vi "Find SGP and PTP.vi"(8 "Error In":errorcluster, 9 "File Path":path, 10 "Pressure, Audio, EGG":dynamicdata(graph)) -> (0 "Error Out":errorcluster, 1 "File Path Indicator":path, 2 "PTP Array":dbl[](array[numeric]), 3 "SGP Array":dbl[](array[numeric]))   [LabVIEW 2018, in "AnalysisSupport.lvlib"]
uses:
  AnalysisSupport.lvlib
  Controls/Intervals.ctl
  <vilib>/Utility/miscctls.llb/LVCursorListTypeDef.ctl
  <vilib>/Waveform/WDTOps.llb/WDT Get XY Value DBL.vi
panel:
  out "PTP":dbl format="%#.3g"
  out "75ms Array":dbl[](array[numeric])
  out "150ms Array":dbl[](array[numeric])
  out "Cutoff (s)":dbl format="%#.3g"
  in  "Show EGG":bool
  in  "Show Audio":bool
  out "File Name":string
  out "End (s)":dbl format="%#.3g"
  out "+75ms":dbl format="%#.3g"
  out "Start (s)":dbl format="%#.3g"
  in  "Undo Button":bool
  in  "Interval (ms)":T1 items=["1000", "500", "330", "250", "150", "50"]
  out "Subset":dynamicdata(graph)
  out "Full Plot":dynamicdata(graph)
  out "Interruptions":i32
  out "SGP":dbl format="%#.3g"
  in  "Okay":bool
  in  "Mark Pressure":bool
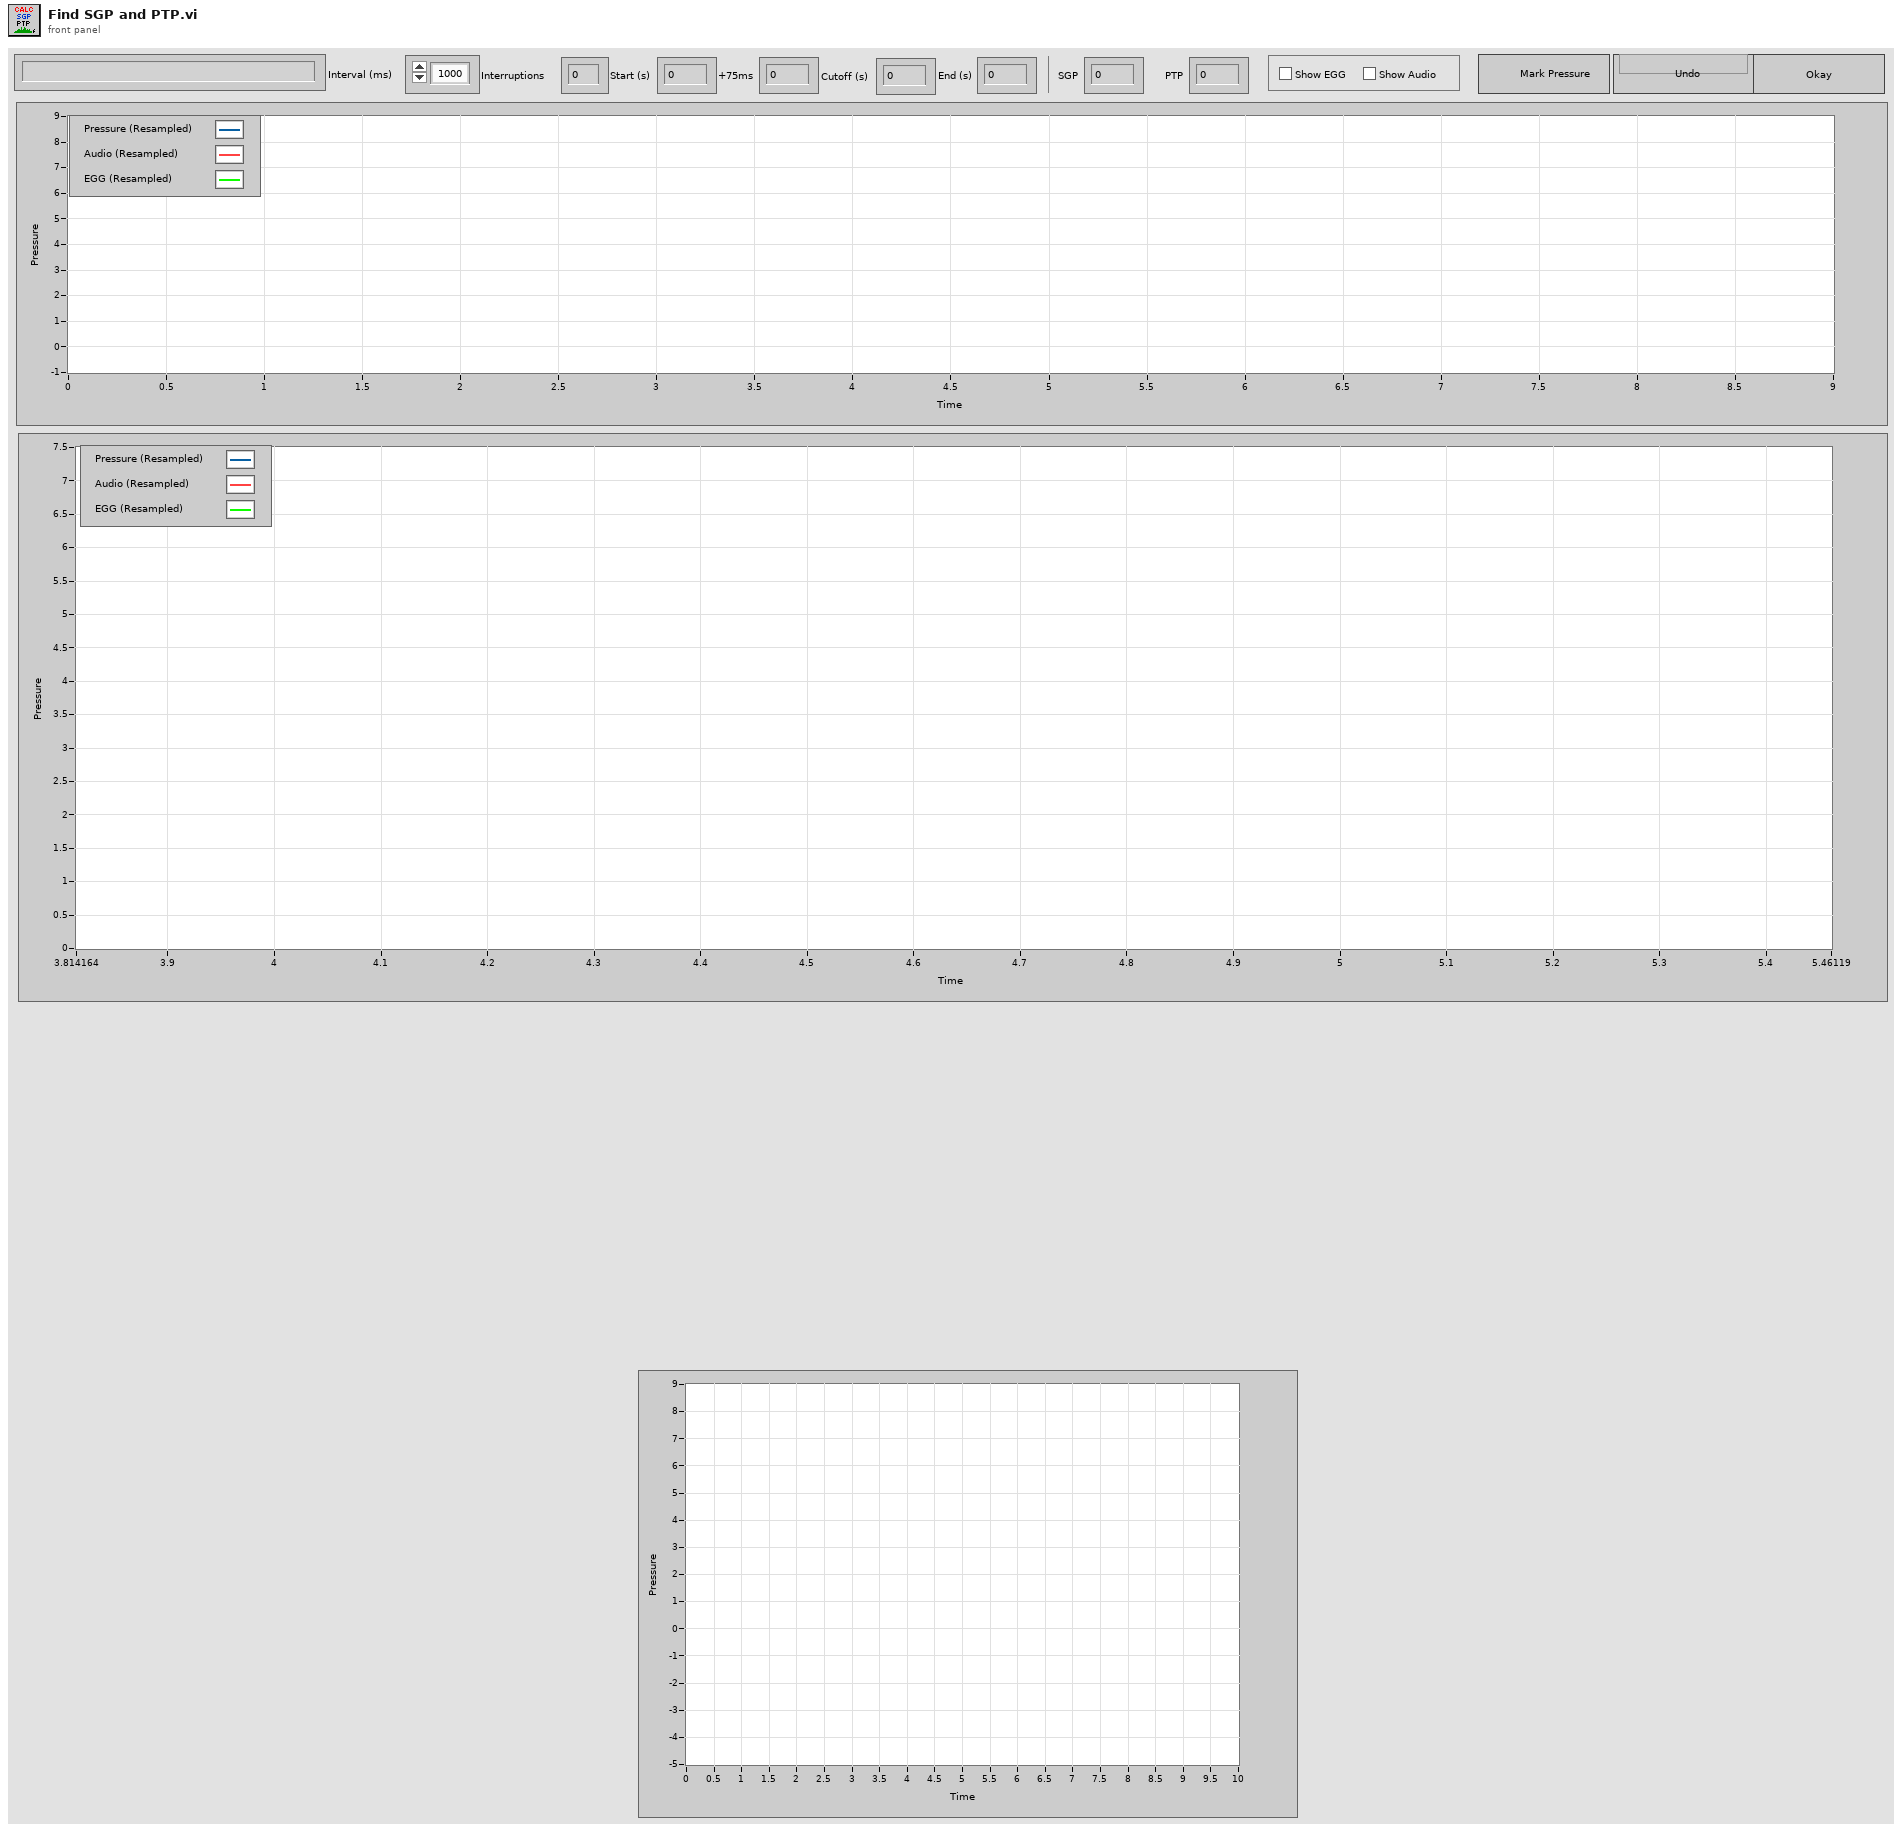
[diagram p1: front panel]
types:
  T1 = typedef "AnalysisSupport.lvlib/Intervals.ctl" = u16
  T2 = typedef "LVCursorListTypeDef.ctl" = cluster{"Name":string, "Color":u32, "Style":u8, "Point Style":u8, "Name Visible":bool, "Allow Drag":bool, "Cursor Mode":u32, "Plot":i32, "Index":i32, "Position":cluster{"X":dbl, "Y":dbl}, "X Scale":u32, "Y Scale":u32, "Watch Plots":i32[], "Watch All Plots":bool, "Plot Area":i32, "Label Offset":cluster{"X":dbl, "Y":dbl}}[]
  T3 = cluster{"Cursor List[0]":cluster{"Name":string, "Color":u32, "Style":u8, "Point Style":u8, "Name Visible":bool, "Allow Drag":bool, "Cursor Mode":u32, "Plot":i32, "Index":i32, "Position":cluster{"X":dbl, "Y":dbl}, "X Scale":u32, "Y Scale":u32, "Watch Plots":i32[], "Watch All Plots":bool, "Plot Area":i32, "Label Offset":cluster{"X":dbl, "Y":dbl}}, "Cursor List[1]":cluster{"Name":string, "Color":u32, "Style":u8, "Point Style":u8, "Name Visible":bool, "Allow Drag":bool, "Cursor Mode":u32, "Plot":i32, "Index":i32, "Position":cluster{"X":dbl, "Y":dbl}, "X Scale":u32, "Y Scale":u32, "Watch Plots":i32[], "Watch All Plots":bool, "Plot Area":i32, "Label Offset":cluster{"X":dbl, "Y":dbl}}, "Cursor List[2]":cluster{"Name":string, "Color":u32, "Style":u8, "Point Style":u8, "Name Visible":bool, "Allow Drag":bool, "Cursor Mode":u32, "Plot":i32, "Index":i32, "Position":cluster{"X":dbl, "Y":dbl}, "X Scale":u32, "Y Scale":u32, "Watch Plots":i32[], "Watch All Plots":bool, "Plot Area":i32, "Label Offset":cluster{"X":dbl, "Y":dbl}}, "Cursor List[3]":cluster{"Name":string, "Color":u32, "Style":u8, "Point Style":u8, "Name Visible":bool, "Allow Drag":bool, "Cursor Mode":u32, "Plot":i32, "Index":i32, "Position":cluster{"X":dbl, "Y":dbl}, "X Scale":u32, "Y Scale":u32, "Watch Plots":i32[], "Watch All Plots":bool, "Plot Area":i32, "Label Offset":cluster{"X":dbl, "Y":dbl}}, "Cursor List[4]":cluster{"Name":string, "Color":u32, "Style":u8, "Point Style":u8, "Name Visible":bool, "Allow Drag":bool, "Cursor Mode":u32, "Plot":i32, "Index":i32, "Position":cluster{"X":dbl, "Y":dbl}, "X Scale":u32, "Y Scale":u32, "Watch Plots":i32[], "Watch All Plots":bool, "Plot Area":i32, "Label Offset":cluster{"X":dbl, "Y":dbl}}, "Cursor List[5]":cluster{"Name":string, "Color":u32, "Style":u8, "Point Style":u8, "Name Visible":bool, "Allow Drag":bool, "Cursor Mode":u32, "Plot":i32, "Index":i32, "Position":cluster{"X":dbl, "Y":dbl}, "X Scale":u32, "Y Scale":u32, "Watch Plots":i32[], "Watch All Plots":bool, "Plot Area":i32, "Label Offset":cluster{"X":dbl, "Y":dbl}}, "Cursor List[6]":cluster{"Name":string, "Color":u32, "Style":u8, "Point Style":u8, "Name Visible":bool, "Allow Drag":bool, "Cursor Mode":u32, "Plot":i32, "Index":i32, "Position":cluster{"X":dbl, "Y":dbl}, "X Scale":u32, "Y Scale":u32, "Watch Plots":i32[], "Watch All Plots":bool, "Plot Area":i32, "Label Offset":cluster{"X":dbl, "Y":dbl}}, "Cursor List[7]":cluster{"Name":string, "Color":u32, "Style":u8, "Point Style":u8, "Name Visible":bool, "Allow Drag":bool, "Cursor Mode":u32, "Plot":i32, "Index":i32, "Position":cluster{"X":dbl, "Y":dbl}, "X Scale":u32, "Y Scale":u32, "Watch Plots":i32[], "Watch All Plots":bool, "Plot Area":i32, "Label Offset":cluster{"X":dbl, "Y":dbl}}, "Cursor List[8]":cluster{"Name":string, "Color":u32, "Style":u8, "Point Style":u8, "Name Visible":bool, "Allow Drag":bool, "Cursor Mode":u32, "Plot":i32, "Index":i32, "Position":cluster{"X":dbl, "Y":dbl}, "X Scale":u32, "Y Scale":u32, "Watch Plots":i32[], "Watch All Plots":bool, "Plot Area":i32, "Label Offset":cluster{"X":dbl, "Y":dbl}}}
  T4 = cluster{"Name":string, "Color":u32, "Style":u8, "Point Style":u8, "Name Visible":bool, "Allow Drag":bool, "Cursor Mode":u32, "Plot":i32, "Index":i32, "Position":cluster{"X":dbl, "Y":dbl}, "X Scale":u32, "Y Scale":u32, "Watch Plots":i32[], "Watch All Plots":bool, "Plot Area":i32, "Label Offset":cluster{"X":dbl, "Y":dbl}}[]
  T5 = cluster{"CrsrList[0]":cluster{"Name":string, "Color":u32, "Style":u8, "Point Style":u8, "Name Visible":bool, "Allow Drag":bool, "Cursor Mode":u32, "Plot":i32, "Index":i32, "Position":cluster{"X":dbl, "Y":dbl}, "X Scale":u32, "Y Scale":u32, "Watch Plots":i32[], "Watch All Plots":bool, "Plot Area":i32, "Label Offset":cluster{"X":dbl, "Y":dbl}}, "CrsrList[1]":cluster{"Name":string, "Color":u32, "Style":u8, "Point Style":u8, "Name Visible":bool, "Allow Drag":bool, "Cursor Mode":u32, "Plot":i32, "Index":i32, "Position":cluster{"X":dbl, "Y":dbl}, "X Scale":u32, "Y Scale":u32, "Watch Plots":i32[], "Watch All Plots":bool, "Plot Area":i32, "Label Offset":cluster{"X":dbl, "Y":dbl}}, "CrsrList[2]":cluster{"Name":string, "Color":u32, "Style":u8, "Point Style":u8, "Name Visible":bool, "Allow Drag":bool, "Cursor Mode":u32, "Plot":i32, "Index":i32, "Position":cluster{"X":dbl, "Y":dbl}, "X Scale":u32, "Y Scale":u32, "Watch Plots":i32[], "Watch All Plots":bool, "Plot Area":i32, "Label Offset":cluster{"X":dbl, "Y":dbl}}, "CrsrList[3]":cluster{"Name":string, "Color":u32, "Style":u8, "Point Style":u8, "Name Visible":bool, "Allow Drag":bool, "Cursor Mode":u32, "Plot":i32, "Index":i32, "Position":cluster{"X":dbl, "Y":dbl}, "X Scale":u32, "Y Scale":u32, "Watch Plots":i32[], "Watch All Plots":bool, "Plot Area":i32, "Label Offset":cluster{"X":dbl, "Y":dbl}}, "CrsrList[4]":cluster{"Name":string, "Color":u32, "Style":u8, "Point Style":u8, "Name Visible":bool, "Allow Drag":bool, "Cursor Mode":u32, "Plot":i32, "Index":i32, "Position":cluster{"X":dbl, "Y":dbl}, "X Scale":u32, "Y Scale":u32, "Watch Plots":i32[], "Watch All Plots":bool, "Plot Area":i32, "Label Offset":cluster{"X":dbl, "Y":dbl}}, "CrsrList[5]":cluster{"Name":string, "Color":u32, "Style":u8, "Point Style":u8, "Name Visible":bool, "Allow Drag":bool, "Cursor Mode":u32, "Plot":i32, "Index":i32, "Position":cluster{"X":dbl, "Y":dbl}, "X Scale":u32, "Y Scale":u32, "Watch Plots":i32[], "Watch All Plots":bool, "Plot Area":i32, "Label Offset":cluster{"X":dbl, "Y":dbl}}, "CrsrList[6]":cluster{"Name":string, "Color":u32, "Style":u8, "Point Style":u8, "Name Visible":bool, "Allow Drag":bool, "Cursor Mode":u32, "Plot":i32, "Index":i32, "Position":cluster{"X":dbl, "Y":dbl}, "X Scale":u32, "Y Scale":u32, "Watch Plots":i32[], "Watch All Plots":bool, "Plot Area":i32, "Label Offset":cluster{"X":dbl, "Y":dbl}}, "CrsrList[7]":cluster{"Name":string, "Color":u32, "Style":u8, "Point Style":u8, "Name Visible":bool, "Allow Drag":bool, "Cursor Mode":u32, "Plot":i32, "Index":i32, "Position":cluster{"X":dbl, "Y":dbl}, "X Scale":u32, "Y Scale":u32, "Watch Plots":i32[], "Watch All Plots":bool, "Plot Area":i32, "Label Offset":cluster{"X":dbl, "Y":dbl}}, "CrsrList[8]":cluster{"Name":string, "Color":u32, "Style":u8, "Point Style":u8, "Name Visible":bool, "Allow Drag":bool, "Cursor Mode":u32, "Plot":i32, "Index":i32, "Position":cluster{"X":dbl, "Y":dbl}, "X Scale":u32, "Y Scale":u32, "Watch Plots":i32[], "Watch All Plots":bool, "Plot Area":i32, "Label Offset":cluster{"X":dbl, "Y":dbl}}}
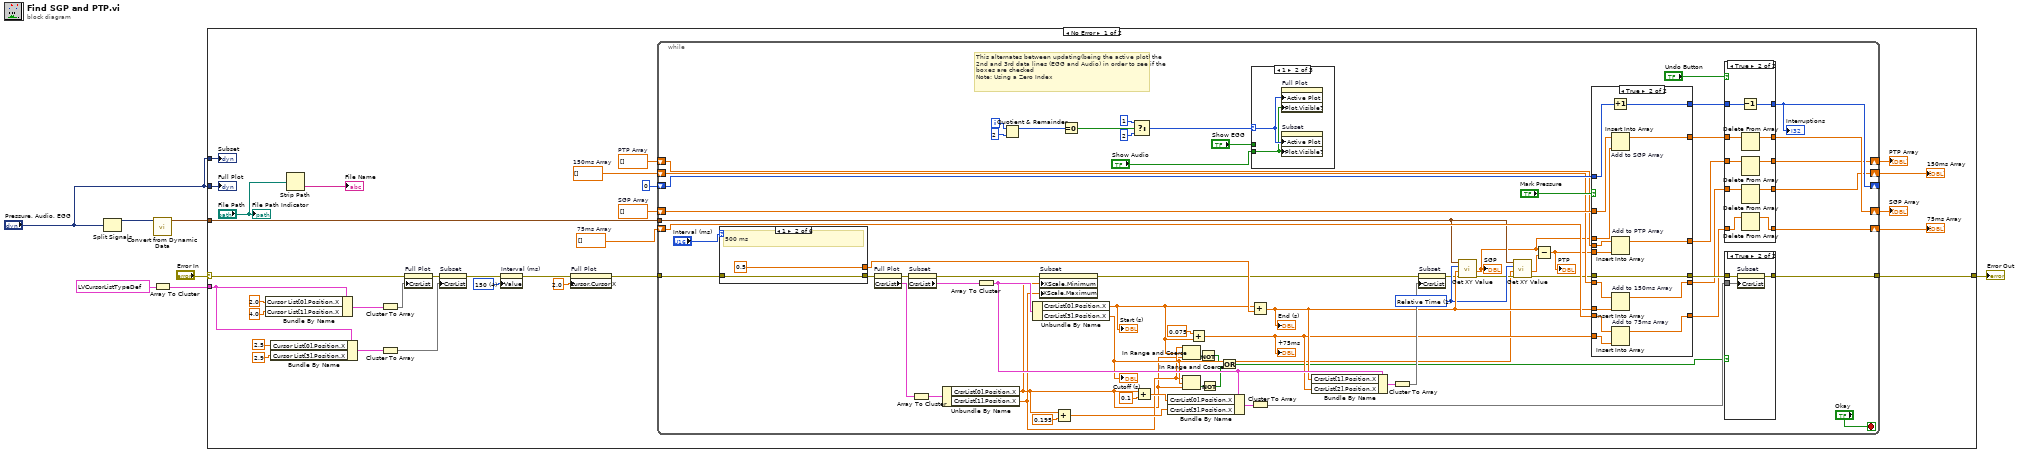
[diagram p0: block diagram]
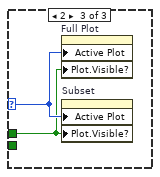
[diagram p3: hidden frame]
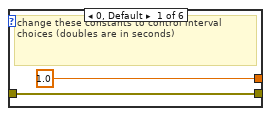
[diagram p5: hidden frame]
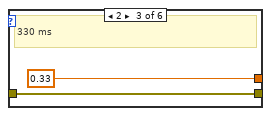
[diagram p6: hidden frame]
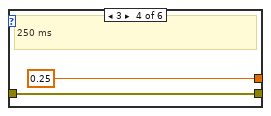
[diagram p7: hidden frame]
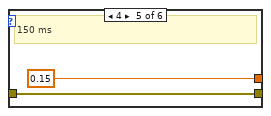
[diagram p8: hidden frame]
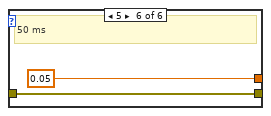
[diagram p9: hidden frame]
diagram:
  n1 = Split Signals("Pressure, Audio, EGG") -> (w2:dynamicdata)  [unwired: 3 in, 2 out]
  n2 = call "Convert from Dynamic Data"("Dynamic Data Type"=w2) -> ("Waveform"=w5:waveform(dbl))  [unwired: 3 in]
  n3 = Array To Cluster(array=T2 [{"Name"="L", "Color"=9843450, "Style"=2, "Point Style"=1, "Name Visible"=FALSE, "Allow Drag"=TRUE, "Cursor Mode"=0, "Plot"=0, "Index"=0, "Position"={"X"=3.0, "Y"=0.0}, "X Scale"=0, "Y Scale"=0, "Watch Plots"=[], "Watch All Plots"=FALSE, "Plot Area"=0, "Label Offset"={"X"=0.0, "Y"=0.0}}, {"Name"="R", "Color"=681210, "Style"=2, "Point Style"=1, "Name Visible"=FALSE, "Allow Drag"=TRUE, "Cursor Mode"=0, "Plot"=0, "Index"=0, "Position"={"X"=-5.0, "Y"=0.0}, "X Scale"=0, "Y Scale"=0, "Watch Plots"=[], "Watch All Plots"=FALSE, "Plot Area"=0, "Label Offset"={"X"=0.0, "Y"=0.0}}, {"Name"="75", "Color"=10174212, "Style"=2, "Point Style"=1, "Name Visible"=FALSE, "Allow Drag"=TRUE, "Cursor Mode"=0, "Plot"=0, "Index"=0, "Position"={"X"=0.0, "Y"=0.0}, "X Scale"=0, "Y Scale"=0, "Watch Plots"=[], "Watch All Plots"=FALSE, "Plot Area"=0, "Label Offset"={"X"=0.0, "Y"=0.0}}, {"Name"="PTP", "Color"=1075712, "Style"=2, "Point Style"=1, "Name Visible"=FALSE, "Allow Drag"=TRUE, "Cursor Mode"=0, "Plot"=0, "Index"=0, "Position"={"X"=0.0, "Y"=0.0}, "X Scale"=0, "Y Scale"=0, "Watch Plots"=[], "Watch All Plots"=FALSE, "Plot Area"=0, "Label Offset"={"X"=0.0, "Y"=0.0}}] ("Cursor List")) -> (cluster=w3:T3)
  n4 = case shown="No Error" "Error In" {
    selector: "Error In" -> [w20 w163]
    tunnel: [w38 w163] -> w7
    tunnel: "Pressure, Audio, EGG" -> [w33 _]
    tunnel: "Pressure, Audio, EGG" -> [w35 _]
    tunnel: w5 -> [w34 _]
    tunnel: w3 -> [w24 _]
    frame No Error {
      w9 = dbl[] []  # PTP Array
      w14 = dbl[] []  # 150ms Array
      w15 = dbl[] []  # 75ms Array
      w18 = T1 4 items=["1000", "500", "330", "250", "150", "50"] ("Interval (ms)")
      w31 = dbl[] []  # SGP Array
      n5 = Bundle By Name(cluster=w24, "Cursor List[0].Position.X"=2.0, "Cursor List[1].Position.X"=4.0) -> (w27:T3)
      n6 = Bundle By Name(cluster=w24, "Cursor List[0].Position.X"=2.5, "Cursor List[3].Position.X"=2.9 ("Cursor List[0].Position.Y")) -> (w22:T3)
      n7 = Strip Path(path="File Path") -> (name=→"File Name":string)  [unwired: 1 out]
      n8 = Cluster To Array(cluster=w27) -> (array=w28:T4)
      n9 = Cluster To Array(cluster=w22) -> (array=w21:T4)
      n10 = property on="Full Plot" class="WFGraph (strict)"(error in=w20, "CrsrList"=w28) -> (error out=w29:errorcluster)  [unwired: 1 in, 1 out]
      n11 = property on="Subset" class="WFGraph (strict)"(error in=w29, "CrsrList"=w21) -> (error out=w16:errorcluster)  [unwired: 1 in, 1 out]
      n12 = property on="Interval (ms)" class="Ring (strict)"(error in=w16, "Value"=w18) -> (error out=w17:errorcluster)  [unwired: 1 in, 1 out]
      n13 = property on="Full Plot" class="WFGraph (strict)"(error in=w17, "Cursor.Cursor X"=2.0 ("Cursor.Cursor Position:Cursor X")) -> (error out=w36:errorcluster)  [unwired: 1 in, 1 out]
      n14 = while {
        tunnel: [w96] -> w38
        tunnel: w36 -> [w92]
        tunnel: w34 -> [w60]
        shift-right: [w81] -> _
        shift-left: 0 -> [w106]
        shift-right: [w79] -> w30
        shift-left: w31 -> [w103]
        shift-right: [w62] -> w10
        shift-left: w15 -> [w78]
        shift-right: [w64] -> w11
        shift-left: w14 -> [w76]
        shift-right: [w51] -> w8
        shift-left: w9 -> [w55]
        i -> [w61]
        stop <- "Okay" stop-if-true
        w59 = u16 1 items=["Samples", "Relative Time"] ("Y position format")
        # "This alternates between updating(being the active plot) the 2nd and 3rd data lines (EGG and Audio) in order to see if the boxes are checked\nNote: Using a Zero Index"
        n15 = case shown="1" "Interval (ms)" {
          tunnel: [w127 w129 w131 w133 w134 w137] -> w91
          tunnel: w92 -> [w127 w129 w131 w133 w134 w137]
          tunnel: [1.0 ("CrsrList[0].Position.X") 0.5 ("CrsrList[0].Position.X") 0.33 ("CrsrList[0].Position.X") 0.25 ("CrsrList[0].Position.X") 0.15 ("CrsrList[0].Position.X") 0.05 ("CrsrList[0].Position.X")] -> w90
          frame 0, Default {
            # "change these constants to control interval choices (doubles are in seconds)"
          }
          frame 1 {
            # "500 ms"
          }
          frame 2 {
            # "330 ms"
          }
          frame 3 {
            # "250 ms"
          }
          frame 4 {
            # "150 ms"
          }
          frame 5 {
            # "50 ms"
          }
        }
        n16 = property on="Full Plot" class="WFGraph (strict)"(error in=w91) -> (error out=w102:errorcluster, "CrsrList"=w99:T2)  [unwired: 1 in, 1 out]
        n17 = property on="Subset" class="WFGraph (strict)"(error in=w102) -> (error out=w101:errorcluster, "CrsrList"=w98:T2)  [unwired: 1 in, 1 out]
        n18 = Array To Cluster(array=w99) -> (cluster=w100:T5)
        n19 = Unbundle By Name(w100) -> ("CrsrList[0].Position.X"=w43:dbl, "CrsrList[1].Position.X"=w44:dbl)
        n20 = Array To Cluster(array=w98) -> (cluster=w88:T5)
        n21 = Quotient & Remainder(x=w61, y=2) -> (x-y*floor(x/y)=w72:i32)  [unwired: 1 out]
        n22 = Unbundle By Name(w88) -> ("CrsrList[0].Position.X"=w46:dbl, "CrsrList[3].Position.X"=w45:dbl)
        "Start (s)" <- w46
        "Cutoff (s)" <- w45
        n23 = property on="Subset" class="WFGraph (strict)"(error in=w101, "XScale.Minimum"=w43, "XScale.Maximum"=w44) -> (error out=w89:errorcluster)  [unwired: 1 in, 1 out]
        n24 = Add(x=w43, y=0.195) -> (x+y=w48:dbl)
        n25 = Equal To 0?(x=w72) -> (x = 0?=w71:bool)
        n26 = Select(t=u32 1 ("Active Plot"), s=w71, f=u32 2 ("Active Plot")) -> (s? t:f=w68:u32)
        n27 = Add(x=w43, y=0.1) -> (x+y=w84:dbl)
        n28 = Bundle By Name(cluster=w88, "CrsrList[0].Position.X"=w84, "CrsrList[3].Position.X"=w48) -> (w95:T5)
        n29 = In Range and Coerce(upper limit=w44, x=w46, lower limit=w43) -> (In Range?=w41:bool)  [unwired: 1 out]
        n30 = In Range and Coerce(upper limit=w44, x=w45, lower limit=w43) -> (In Range?=w42:bool)  [unwired: 1 out]
        n31 = Add(x=0.075, y=w46) -> (x+y=w74:dbl)
        "+75ms" <- w74
        n32 = Not(x=w41) -> (.not. x?=w40:bool)
        n33 = Not(x=w42) -> (.not. x?=w39:bool)
        n34 = Or(x=w40, y=w39) -> (x .or. y?=w47:bool)
        n35 = case shown="1" w68 {
          selector: w68 -> [_ w108 w110]
          tunnel: "Show Audio" -> [_ w107 _]
          tunnel: "Show EGG" -> [_ _ w109]
          frame 0, Default {
          }
          frame 1 {
            n36 = property on="Full Plot" class="WFGraph (strict)"("Active Plot"=w108, "Plot.Visible?"=w107) -> ()  [unwired: 2 in, 2 out]
            n37 = property on="Subset" class="WFGraph (strict)"("Active Plot"=w108, "Plot.Visible?"=w107) -> ()  [unwired: 2 in, 2 out]
          }
          frame 2 {
            n38 = property on="Full Plot" class="WFGraph (strict)"("Active Plot"=w110, "Plot.Visible?"=w109) -> ()  [unwired: 2 in, 2 out]
            n39 = property on="Subset" class="WFGraph (strict)"("Active Plot"=w110, "Plot.Visible?"=w109) -> ()  [unwired: 2 in, 2 out]
          }
        }
        n40 = Add(x=w46, y=w90) -> (x+y=w75:dbl)
        "End (s)" <- w75
        n41 = Cluster To Array(cluster=w95) -> (array=w94:T4)
        n42 = Bundle By Name(cluster=w88, "CrsrList[1].Position.X"=w75, "CrsrList[2].Position.X"=w74) -> (w87:T5)
        n43 = Cluster To Array(cluster=w87) -> (array=w86:T4)
        n44 = property on="Subset" class="WFGraph (strict)"(error in=w89, "CrsrList"=w86) -> (error out=w58:errorcluster)  [unwired: 1 in, 1 out]
        n45 = call-poly <vilib>:"Get XY Value.vi"("error in (no error)"=w58, "Y position"=w75, "Y position format"=w59, "waveform in"=w60) -> ("error out"=w57:errorcluster, "Y value"=w53:dbl)  [unwired: 3 in, 3 out]
        "SGP" <- w53
        n46 = call-poly <vilib>:"Get XY Value.vi"("error in (no error)"=w57, "Y position"=w45, "Y position format"=w59, "waveform in"=w60) -> ("error out"=w56:errorcluster, "Y value"=w52:dbl)  [unwired: 3 in, 3 out]
        n47 = Subtract(x=w53, y=w52) -> (x-y=w50:dbl)
        "PTP" <- w50
        n48 = case shown="True" "Mark Pressure" {
          tunnel: w56 -> [w147 w162]
          tunnel: [w147 w162] -> w97
          tunnel: w106 -> [w146 w157]
          tunnel: [w146 w161] -> w82
          tunnel: w53 -> [_ w158]
          tunnel: w103 -> [w145 w160]
          tunnel: [w145 w159] -> w80
          tunnel: w78 -> [w144 w156]
          tunnel: [w144 w155] -> w63
          tunnel: w74 -> [_ w154]
          tunnel: w76 -> [w143 w153]
          tunnel: w75 -> [_ w152]
          tunnel: [w143 w151] -> w65
          tunnel: w55 -> [w142 w149]
          tunnel: [w142 w150] -> w54
          tunnel: w50 -> [_ w148]
          frame False {
          }
          frame True {
            n49 = Increment(x=w157) -> (x+1=w161:i32)
            n50 = Insert Into Array "Add to SGP Array"(array=w160, new element=w158) -> (w159:dbl[])  [unwired: 1 in]
            n51 = Insert Into Array "Add to PTP Array"(array=w149, new element=w148) -> (w150:dbl[])  [unwired: 1 in]
            n52 = Insert Into Array "Add to 150ms Array"(array=w153, new element=w152) -> (w151:dbl[])  [unwired: 1 in]
            n53 = Insert Into Array "Add to 75ms Array"(array=w156, new element=w154) -> (w155:dbl[])  [unwired: 1 in]
          }
        }
        n54 = case shown="True" "Undo Button" {
          tunnel: w80 -> [w115 w125]
          tunnel: [w115 w124] -> w79
          tunnel: w82 -> [w114 w123]
          tunnel: [w114 w122] -> w81
          tunnel: w65 -> [w113 w121]
          tunnel: [w113 w120] -> w64
          tunnel: w63 -> [w112 w119]
          tunnel: [w112 w118] -> w62
          tunnel: w54 -> [w111 w117]
          tunnel: [w111 w116] -> w51
          frame False {
          }
          frame True {
            n55 = Decrement(x=w123) -> (x-1=w122:i32)
            n56 = Delete From Array(array=w125) -> (array with subset deleted=w124:dbl[])  [unwired: 2 in, 1 out]
            n57 = Delete From Array(array=w117) -> (array with subset deleted=w116:dbl[])  [unwired: 2 in, 1 out]
            n58 = Delete From Array(array=w121) -> (array with subset deleted=w120:dbl[])  [unwired: 2 in, 1 out]
            n59 = Delete From Array(array=w119) -> (array with subset deleted=w118:dbl[])  [unwired: 2 in, 1 out]
          }
        }
        "Interruptions" <- w81
        n60 = case shown="True" w47 {
          tunnel: w97 -> [w138 w141]
          tunnel: [w138 w140] -> w96
          tunnel: w94 -> [_ w139]
          frame False {
          }
          frame True {
            n61 = property on="Subset" class="WFGraph (strict)"(error in=w141, "CrsrList"=w139) -> (error out=w140:errorcluster)  [unwired: 1 in, 1 out]
          }
        }
      }
      "SGP Array" <- w30
      "150ms Array" <- w11
      "75ms Array" <- w10
      "PTP Array" <- w8
      "File Path Indicator" <- "File Path"
      "Subset" <- w35
      "Full Plot" <- w33
    }
    frame Error {
    }
  }
  "Error Out" <- w7
